vi "p2.4 (hw1).vi"() -> ()   [LabVIEW 2017]
panel:
  out "Output F(x)":dbl
  in  "Input":dbl
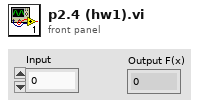
[diagram p1: front panel]
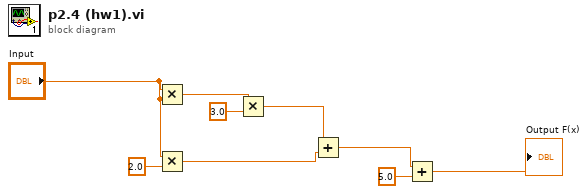
[diagram p0: block diagram]
diagram:
  n1 = Multiply(x="Input", y="Input") -> (x*y=w9:dbl)
  n2 = Multiply(x="Input", y=2.0) -> (x*y=w4:dbl)
  n3 = Multiply(x=w9, y=3.0) -> (x*y=w5:dbl)
  n4 = Add(x=w5, y=w4) -> (x+y=w3:dbl)
  n5 = Add(x=w3, y=5.0) -> (x+y=→"Output F(x)":dbl)
